vi "digitalOut.vi"(9 "rate":dbl=10000.0 format="%#_13g", 10 "waveform":bool[][](array[boolean]), 11 "lines":tag="cDAQ9185-1D03A69Mod3/port0/line0:4") -> (2 "digital waveform":digitalwaveform(waveform)={"t0"=timestamp(0 s since 1904-01-01), "dt"=0.0, "Y"={"transitions"=[], "data"=[]}, "error"={"status"=FALSE, "code"=37421928, "source"=""}})   [LabVIEW 2017]
uses:
  <vilib>/DAQmx/write.llb/DAQmx Write (Digital 2D U8 NChan NSamp).vi
  <vilib>/DAQmx/create/channels.llb/DAQmx Create Channel (DO-Digital Output).vi
  <vilib>/DAQmx/configure/timing.llb/DAQmx Timing (Sample Clock).vi
  <vilib>/Waveform/DWDTOps.llb/DWDT Boolean Array to Digital.vi
  <vilib>/Waveform/DWDTOps.llb/DWDT Digital to Binary U8.vi
  <vilib>/DAQmx/miscellaneous.llb/DAQmx Fill In Error Info.vi
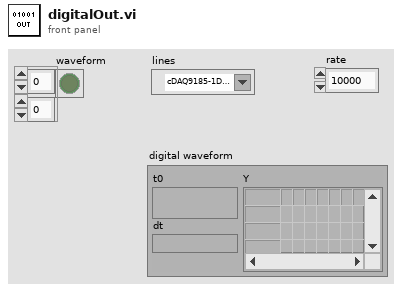
[diagram p1: front panel]
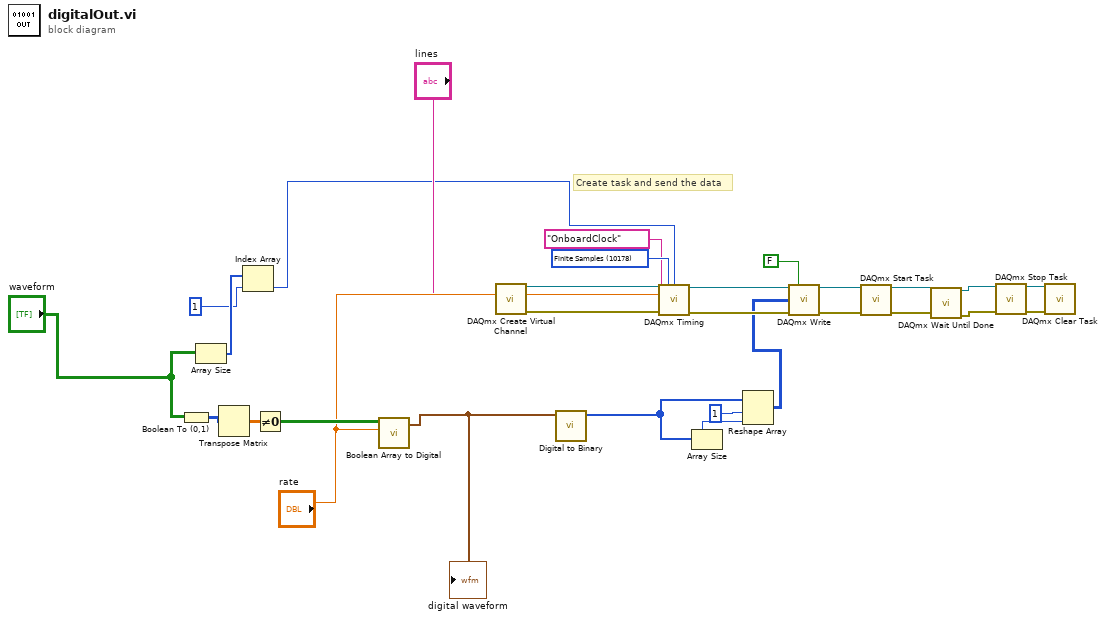
[diagram p0: block diagram]
diagram:
  w11 = 10178 items=["Finite Samples"=10178, "Continuous Samples"=10123, "Hardware Timed Single Point"=12522] ("sample mode")
  # "Create task and send the data"
  n1 = Boolean To (0,1)(Boolean="waveform") -> (0, 1=w29:i16[][])
  n2 = Array Size(array="waveform") -> (size(s)=w9:i32[])
  n3 = Transpose Matrix(1:w29) -> (0:w28:dbl[][])
  n4 = Index Array(array=w9, index=1) -> (element=w6:i32)
  n5 = Not Equal To 0?(x=w28) -> (x != 0?=w27:bool[][])
  n6 = call-poly <vilib>:"Boolean Array to Digital.vi"("sample rate"="rate", "boolean array"=w27) -> ("digital waveform"=w21:digitalwaveform)  [unwired: 8 in, 1 out]
  "digital waveform" <- w21
  n7 = call-poly <vilib>:"DAQmx Create Virtual Channel.vi"("lines"="lines") -> ("task out"=w26:refnum<k21>, "error out"=w25:errorcluster)  [unwired: 13 in]
  n8 = call-poly <vilib>:"Digital to Binary.vi"("digital waveform"=w21) -> ("binary array"=w18:u8[])  [unwired: 9 in, 1 out]
  n9 = call-poly <vilib>:"DAQmx Timing.vi"("task/channels in"=w26, "sample mode"=w11, "samples per channel"=w6, "rate"="rate", "source"=tag "OnboardClock", "error in"=w25) -> ("task out"=w24:refnum<k21>, "error out"=w23:errorcluster)  [unwired: 8 in]
  n10 = Array Size(array=w18) -> (size(s)=w17:i32)
  n11 = Reshape Array(w18, 1, w17) -> (w19:u8[][])
  n12 = call-poly <vilib>:"DAQmx Write.vi"("task/channels in"=w24, "auto start"=FALSE, "data"=w19, "error in"=w23) -> ("task out"=w16:refnum<k21>, "error out"=w15:errorcluster)  [unwired: 9 in, 1 out]
  n13 = call <vilib>:"DAQmx Start Task.vi"("task/channels in"=w16, "error in"=w15) -> ("task out"=w5:refnum<k21>, "error out"=w4:errorcluster)  [unwired: 12 in]
  n14 = call <vilib>:"DAQmx Wait Until Done.vi"("task/channels in"=w5, "error in"=w4) -> ("task out"=w3:refnum<k21>, "error out"=w2:errorcluster)  [unwired: 12 in]
  n15 = call <vilib>:"DAQmx Stop Task.vi"("task/channels in"=w3, "error in"=w2) -> ("task out"=w14:refnum<k21>, "error out"=w13:errorcluster)  [unwired: 12 in]
  n16 = call <vilib>:"DAQmx Clear Task.vi"("task in"=w14, "error in"=w13) -> ()  [unwired: 13 in, 1 out]
